vi "表格控件.vi"() -> ()   [LabVIEW 2010]
uses:
  Instance           1 16Saved   表格控件 .vi
  <vilib>/measure/NI_MABase.lvlib
panel:
  out "表格":string[][](table)
  out "表格控件":string[][](table)=[["0.3913", "0.4278", "0.0800", "0.1502", "0.6405", "0.1857", "0.6750", "0.3588", "0.8628", "0.9539"], ["0.6780", "0.6843", "0.0183", "0.0632", "0.7202", "0.9063", "0.0268", "0.8160", "0.3780", "0.8213"], ["0.8182", "0.8767", "0.2896", "0.3767", "0.9318", "0.7983", "0.1455", "0.1253", "0.4073", "0.6418"], ["0.7434", "0.8939", "0.4911", "0.7317", "0.3892", "0.2635", "0.1266", "0.8595", "0.0673", "0.6548"], ["0.7692", "0.3098", "0.4323", "0.4352", "0.7735", "0.0667", "0.5172", "0.4932", "0.1523", "0.3084"], ["0.2725", "0.1220", "0.7000", "0.8563", "0.4687", "0.5576", "0.0084", "0.7922", "0.8546", "0.1711"], ["0.4876", "0.6553", "0.6199", "0.7224", "0.7569", "0.8251", "0.8462", "0.8473", "0.7745", "0.3654"], ["0.7665", "0.6694", "0.9915", "0.0186", "0.3264", "0.5071", "0.1996", "0.7507", "0.0200", "0.6615"], ["0.1204", "0.5829", "0.5978", "0.6000", "0.2914", "0.9173", "0.2592", "0.6027", "0.9688", "0.3986"], ["0.9871", "0.6176", "0.9533", "0.8757", "0.4383", "0.5404", "0.5721", "0.5695", "0.9496", "0.5997"]]
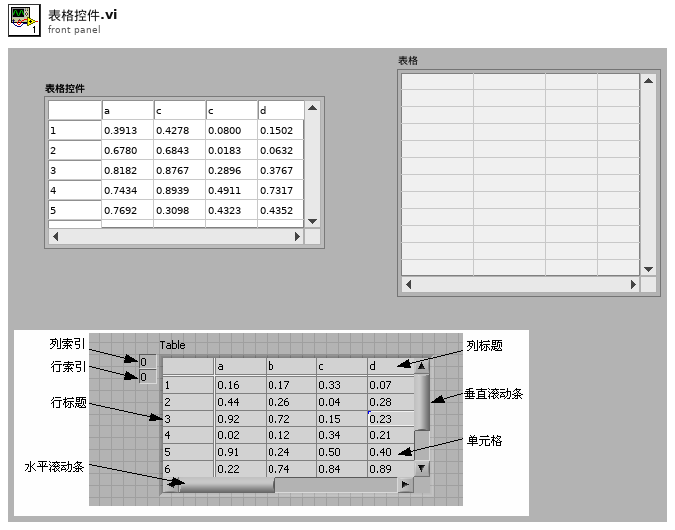
[diagram p1: front panel]
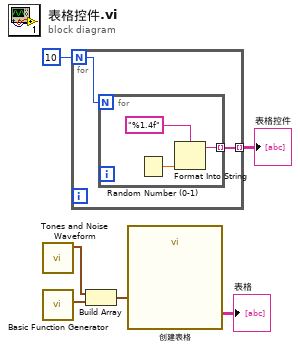
[diagram p0: block diagram]
diagram:
  n1 = call <vilib>:"Tones and Noise Waveform.vi"() -> ("signal out"=w3:waveform(dbl))  [unwired: 10 in, 1 out]
  n2 = call <vilib>:"Basic Function Generator.vi"() -> ("signal out"=w2:waveform(dbl))  [unwired: 9 in, 2 out]
  n3 = for {
    N: 10 -> [w8]
    tunnel: [w7] -> w5 mode=indexing
    n4 = for {
      N: w8 -> [_]
      tunnel: [w11] -> w7 mode=indexing
      n5 = Random Number (0-1)() -> (number: 0 to 1=w9:dbl)
      n6 = Format Into String(format string="%1.4f" ("格式字符串"), w9) -> (resulting string=w11:string)  [unwired: 2 in, 1 out]
    }
  }
  "表格控件" <- w5
  n7 = Build Array(w3, w2) -> (w1:waveform(dbl)[])
  n8 = call "创建表格"("Signals"=w1) -> ("Table"=→"表格":string[][])  [unwired: 9 in, 1 out]
